vi "Apply.vi"(8 "error in":errorcluster, 11 "DO DAQmx PWM Fixed Freq in":refnum<class "DO DAQmx PWM Fixed Freq CFG.lvclass">) -> (0 "error out":errorcluster, 3 "DO DAQmx PWM Fixed Freq out":refnum<class "DO DAQmx PWM Fixed Freq CFG.lvclass">)   [LabVIEW 2023, in "DAQmx Simulated CFGs.lvlib" / "DO DAQmx PWM Fixed Freq CFG.lvclass"]
uses:
  DO DAQmx PWM Fixed Freq CFG.lvclass
  Configuration/Configuration JSON/Configuration JSON Base/CFG JSON.lvclass/CFG JSON.ctl
  DO DAQmx Fixed Freq PWM CFG/DO DAQmx Fixed Freq PWM CFG.lvclass
  DO DAQmx PWM Fixed Freq CFG.lvclass/DO DAQmx PWM Fixed Freq CFG.ctl
  Configuration/Configuration JSON/Configuration JSON Base/CFG JSON.lvclass
  D:/git/HAL/HAL GOOP4/DIO/DO DAQmx Fixed Freq PWM CFG/DO DAQmx Fixed Freq PWM CFG.lvclass
  D:/git/HAL/HAL GOOP4/DAQmx/DAQmx Base CFG/DAQmx Base CFG.lvclass
  D:/git/HAL/HAL GOOP4/CFG Target/CFG Target.lvclass
  D:/git/HAL/HAL GOOP4/Configuration/Configuration Semaphore/CFG Semaphore.lvclass
  D:/git/HAL/HAL GOOP4/Configuration/Configuration JSON/Configuration JSON Base/CFG JSON.lvclass
  D:/git/HAL/HAL GOOP4/Interfaces/IConfigure/IConfigure.lvclass
  D:/git/HAL/HAL GOOP4/DIO/DIO DAQmx Simulated CFGs/DO DAQmx PWM Fixed Freq CFG/DO DAQmx PWM Fixed Freq CFG.lvclass
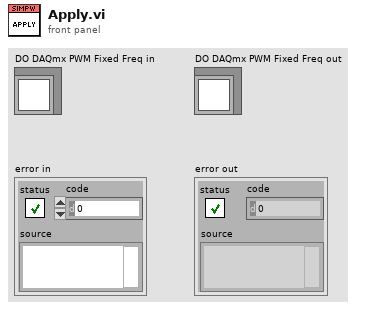
[diagram p1: front panel]
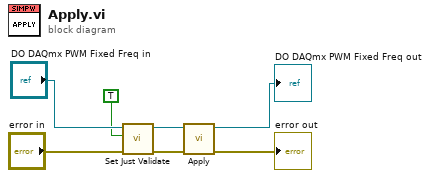
[diagram p0: block diagram]
diagram:
  n1 = call "Set Just Validate.vi"("error in (no error)"="error in", "Just Validate"=TRUE, "CFG JSON Base in"="DO DAQmx PWM Fixed Freq in") -> ("error out"=w4:errorcluster, "CFG JSON Base out"=w2:refnum<class "DO DAQmx PWM Fixed Freq CFG.lvclass">)  [unwired: 7 in]
  n2 = call-parent "Apply.vi"("error in"=w4, "DO DAQmx Fixed Freq PWM CFG in"=w2) -> ("error out"=→"error out":errorcluster, "DO DAQmx Fixed Freq PWM CFG out"=→"DO DAQmx PWM Fixed Freq out":refnum<class "DO DAQmx PWM Fixed Freq CFG.lvclass">)  [unwired: 8 in]
